vi "IMAQ to Array.vi"(8 "error in (no error)":errorcluster, 11 "Refnum in":T1) -> (0 "error out":errorcluster, 3 "Array":u8[][][](array[numeric]))   [LabVIEW 2022 SP3]
uses:
  <vilib>/vision/Image Controls.llb/IMAQ Image.ctl
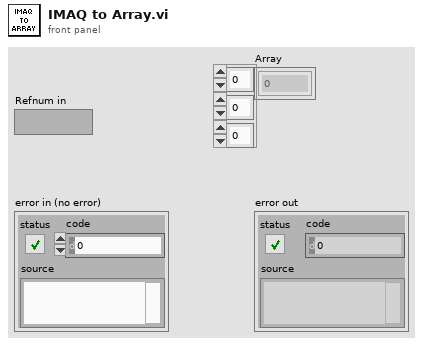
[diagram p1: front panel]
types:
  T1 = typedef "IMAQ Image.ctl" = refnum<image>
  T2 = enum16{"big-endian, network order", "native, host order", "little-endian"}
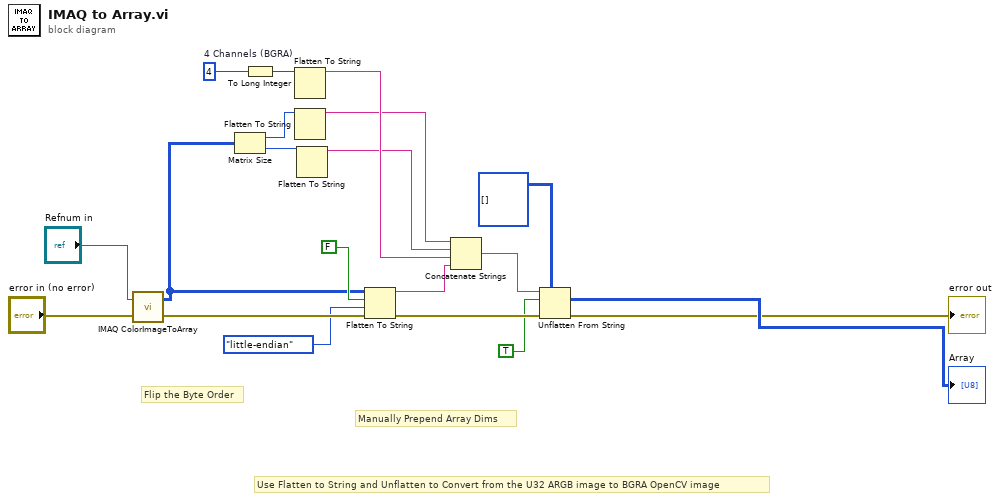
[diagram p0: block diagram]
diagram:
  w9 = 4  # 4 Channels (BGRA)
  # "Use Flatten to String and Unflatten to Convert from the U32 ARGB image to BGRA OpenCV image"
  # "Flip the Byte Order"
  # "Manually Prepend Array Dims"
  n1 = call "IMAQ ColorImageToArray"("Image"="Refnum in", "error in (no error)"="error in (no error)") -> ("Image Pixels (U32)"=w12:u32[][], "error out"=w14:errorcluster)  [unwired: 2 in, 1 out]
  n2 = Matrix Size(0:w12) -> (1:w10:i32, 2:w11:i32)
  n3 = To Long Integer(number=w9) -> (32bit integer=w8:i32)
  n4 = Flatten To String(anything=w8) -> (data string=w3:string)  [unwired: 3 in, 2 out]
  n5 = Flatten To String(anything=w10) -> (data string=w2:string)  [unwired: 3 in, 2 out]
  n6 = Flatten To String(anything=w11) -> (data string=w1:string)  [unwired: 3 in, 2 out]
  n7 = Flatten To String(anything=w12, prepend array or string size? (T)=FALSE, byte order (0:big-endian, network order)=T2."little-endian", error in (no error)=w14) -> (data string=w7:string, error out=w15:errorcluster)  [unwired: 1 out]
  n8 = Concatenate Strings(w2, w1, w3, w7) -> (w6:string)
  n9 = Unflatten From String(type=u8[][][] [] ("Array"), binary string=w6, data includes array or string size? (T)=TRUE, error in (no error)=w15) -> (value=→"Array":u8[][][], error out=→"error out":errorcluster)  [unwired: 1 in, 1 out]
